vi "Main Tclk.vi"() -> ()   [LabVIEW 2018] (continued)
                    n1849 = shared-variable ".\\Zeiss Library.lvlib\\Timestamp"() -> (w7479:timestamp)  [unwired: 1 in, 1 out]
                    n1850 = Unbundle By Name(w7478) -> ("Frames"=w7475:u8, "Y tiles"=w7477:u8, "X tiles"=w7476:u8)
                    n1851 = for {
                      N: w7475 -> [_]
                      tunnel: w7479 -> [w7483]
                      tunnel: w7477 -> [w7482]
                      tunnel: w7476 -> [w7481]
                      i -> [w7480]
                      n1852 = for {
                        N: w7482 -> [_]
                        tunnel: w7481 -> [w7487]
                        tunnel: w7483 -> [w7485]
                        tunnel: w7480 -> [w7484]
                        i -> [w7486]
                        n1853 = for {
                          N: w7487 -> [_]
                          tunnel: w7486 -> [w7494]
                          tunnel: w7485 -> [w7491]
                          tunnel: w7484 -> [w7490]
                          i -> [w7493]
                          w7489 = "-" ("string")
                          w7516 = "^" ("replace string (\"\")")
                          w7496 = "_" ("string")
                          n1854 = local read "Hardware Configuration"() -> (w7526:T25)
                          n1855 = local read "File Information"() -> (w7528:T31)
                          n1856 = Format Into String(w7490) -> (resulting string=w7488:string)  [unwired: 3 in, 1 out]
                          n1857 = Format Into String(w7494) -> (resulting string=w7495:string)  [unwired: 3 in, 1 out]
                          n1858 = Format Into String(w7493) -> (resulting string=w7492:string)  [unwired: 3 in, 1 out]
                          n1859 = Unbundle By Name(w7526) -> ("Machine ID"=w7525:string)
                          n1860 = Format Date/Time String(time format string (%c)="%y-%m-%d_%H%M%S", seconds (now)=w7491) -> (date/time string=w7531:string)  [unwired: 1 out]
                          n1861 = local read "SEM Options"() -> (w7511:T27)
                          n1862 = Unbundle By Name(w7528) -> ("Sample ID"=w7513:string, "File path"=w7527:path)
                          n1863 = Format Date/Time String(time format string (%c)="Y%Y\\M%m\\D%d", seconds (now)=w7491) -> (date/time string=w7536:string)  [unwired: 1 out]
                          n1864 = xnode "Match Regular Expression"("input string"=w7525, "regular expression"="/") -> ("after match"=w7535:string)  [unwired: 4 in, 4 out]
                          n1865 = Concatenate Strings(w7535, w7496, w7531, w7496, w7488, w7489, w7495, w7489, w7492, ".dat" ("string")) -> (w7537:string)
                          n1866 = Unbundle By Name(w7511) -> ("Delete after upload"=w7510:bool)
                          n1867 = Build Path(base path=w7527, name or relative path=w7536) -> (appended path=w7533:path)
                          n1868 = Build Path(base path=w7533, name or relative path=w7537) -> (appended path=w7512:path)
                          n1869 = Path To String(path=w7512) -> (string=w7519:string)
                          n1870 = shared-variable ".\\Zeiss Library.lvlib\\Upload flags path"() -> (w7498:string)  [unwired: 1 in, 1 out]
                          n1871 = Search and Replace String(replace all?=TRUE ("replace all? (F)"), input string=w7519, search string="\\", replace string=w7516) -> (result string=w7515:string)  [unwired: 4 in, 3 out]
                          n1872 = Select(t="^delete" ("replace string (\"\")"), s=w7510, f="^keep" ("replace string (\"\")")) -> (s? t:f=w7524:string)
                          n1873 = Search and Replace String(input string=w7515, search string=":", replace string=w7516) -> (result string=w7520:string)  [unwired: 5 in, 3 out]
                          n1874 = String To Path(string=w7498) -> (path=w7497:path)
                          n1875 = Concatenate Strings(w7513, "^" ("string"), w7520, w7524) -> (w7499:string)
                          n1876 = Build Path(base path=w7497, name or relative path="Filtered") -> (appended path=w7504:path)
                          n1877 = Build Path(base path=w7497, name or relative path=w7499) -> (appended path=w7509:path)
                          n1878 = File/Directory Info(path=w7504) -> (path out=w7502:path, error out=w7503:errorcluster)  [unwired: 1 in, 5 out]
                          n1879 = File/Directory Info(path=w7509) -> (path out=w7508:path, error out=w7507:errorcluster)  [unwired: 1 in, 5 out]
                          n1880 = Unbundle By Name(w7503) -> ("status"=w7501:bool)
                          n1881 = Unbundle By Name(w7507) -> ("status"=w7506:bool)
                          n1882 = case shown="True" w7501 {
                            tunnel: w7502 -> [w7538 w7540]
                            tunnel: [w7538 w7539] -> w7500
                            frame False {
                            }
                            frame True {
                              n1883 = Create Folder(path (use dialog)=w7540) -> (created path=w7539:path)  [unwired: 2 in, 2 out]
                            }
                          }
                          n1884 = case shown="False" w7506 {
                            tunnel: w7508 -> [w7544 _]
                            tunnel: w7500 -> [w7542 _]
                            tunnel: w7499 -> [w7541 _]
                            frame False {
                              n1885 = Build Path(base path=w7542, name or relative path=w7541) -> (appended path=w7543:path)
                              n1886 = Move(source path=w7544, 10:w7543) -> ()  [unwired: 3 in, 3 out]
                            }
                            frame True {
                            }
                          }
                        }
                      }
                    }
                  }
                }
                n1887 = local write "Milling Z voltage array"(w7470) -> ()
                n1888 = Array Size(array=w7470) -> (size(s)=w7445:i32)
                n1889 = Subtract(x=w7445, y=w7444) -> (x-y=w7469:i32)
                n1890 = Max & Min(x=w7445, y=w7444) -> (min(x,y)=w7446:i32)  [unwired: 1 out]
                n1891 = Array Subset(array=w7470, index=w7469, length=w7446) -> (w7471:sgl[])
                n1892 = for {
                  N: w7446 -> [_]
                  tunnel: [w7474] -> w7447 mode=indexing
                  i -> [w7474]
                }
                n1893 = call <vilib>:"Linear Fit.vi"("Y"=w7471, "X"=w7447) -> ("slope"=w7466:dbl)  [unwired: 9 in, 4 out]
                n1894 = local read "Milling para"() -> (w7464:T35)
                n1895 = local read "FIB Scan Parameters"() -> (w7467:T32)
                n1896 = Greater Or Equal?(x=w7445, y=100.0) -> (x >= y?=w7458:bool)
                n1897 = Unbundle By Name(w7464) -> ("FIB FOV (um)"=w7463:sgl)
                n1898 = Unbundle By Name(w7467) -> ("Z size (V)"=w7465:dbl)
                n1899 = Select(t=T44."Enabled" ("Disabled"), s=w7458, f=T44."Disabled and Grayed Out" ("Disabled")) -> (s? t:f=w7457:T44)
                n1900 = Divide(x=w7466, y=w7465) -> (x/y=w7462:dbl)
                n1901 = Compound Arithmetic op=MULTIPLY(w7463, sgl -1000.0 ("value"), w7462) -> (w7452:dbl)
                "Delta Z (nm)" <- w7452
                n1902 = property on="Delta Z (nm)" class="DigNum (strict)"("DisabledEnum"=w7457) -> ()  [unwired: 2 in, 2 out]
                n1903 = local read "Delta Z array"() -> (w7454:sgl[])
                n1904 = local read "SEM Specimen I array"() -> (w7456:sgl[])
                n1905 = local read "SEM Specimen I"() -> (w7423:dbl)
                n1906 = Build Array (concatenate)(w7454, w7452) -> (w7453:dbl[])
                n1907 = local write "Delta Z array"(w7453) -> ()
                n1908 = Build Array (concatenate)(w7456, w7423) -> (w7455:dbl[])
                n1909 = local write "SEM Specimen I array"(w7455) -> ()
                n1910 = local read "3D FIB-SEM Files"() -> (w7427:path)
                n1911 = local read "SEM Scan Parameters"() -> (w7432:T26)
                n1912 = Unbundle By Name(w7432) -> ("Y tiles"=w7435:u8, "X tiles"=w7433:u8)
                n1913 = Build Array(w7435, w7433) -> (w7434:u8[])
                n1914 = Quotient & Remainder(x=w7434, y=2) -> (floor(x/y)=w7430:i32[])  [unwired: 1 out]
                n1915 = Index Array(array=w7430) -> (element #1=w7441:i32, element #2=w7442:i32)  [unwired: 2 in]
                n1916 = Format Into String(w7441) -> (resulting string=w7440:string)  [unwired: 3 in, 1 out]
                n1917 = Format Into String(w7442) -> (resulting string=w7438:string)  [unwired: 3 in, 1 out]
                n1918 = Concatenate Strings("Low res_" ("string"), w7440, "-" ("string"), w7438, ".png" ("string")) -> (w7429:string)
                n1919 = Build Path(base path=w7427, name or relative path=w7429) -> (appended path=w7426:path)
                n1920 = Build Path(base path=w7427, name or relative path="Low res.png" ("string")) -> (appended path=w7425:path)
                n1921 = Copy(9:TRUE ("overwrite (F)"), 10:w7425, 11:w7426) -> ()  [unwired: 2 in, 3 out]
              }
              frame #24 {
                n1922 = local read "SEM Scan Parameters"() -> (w7668:T26)
                n1923 = local read "Auto re-engage"() -> (w7669:bool)
                n1924 = local read "Reheat from last"() -> (w7665:bool)
                n1925 = Unbundle By Name(w7668) -> ("Pixel size (nm)"=w7667:sgl, "Y tiles"=w7661:u8, "X tiles"=w7660:u8)
                n1926 = expression code="x/1000"(w7667) -> (w7666:sgl)
                n1927 = Build Array(w7661, w7660) -> (w7663:u8[])
                n1928 = Quotient & Remainder(x=w7663, y=2) -> (floor(x/y)=w7656:i32[])  [unwired: 1 out]
                n1929 = Index Array(array=w7656) -> (element #1=w7659:i32, element #2=w7658:i32)  [unwired: 2 in]
                n1930 = local read "Low res scale tiled"() -> (w7664:dbl[][])
                n1931 = Index Array(array=w7664, index (row)=w7659, index (col)=w7658) -> (element=w7657:dbl)
                n1932 = case shown="False" w7669 {
                  tunnel: w7666 -> [_ w7714]
                  tunnel: w7657 -> [_ w7713]
                  frame False {
                    n1933 = local read "Re-engage counts"() -> (w7689:u8)
                    n1934 = local read "Last re-engage count"() -> (w7691:u8)
                    n1935 = Less?(x=w7689, y=w7691) -> (x < y?=w7690:bool)
                    n1936 = case shown="True" w7690 {
                      tunnel: w7689 -> [_ w7700]
                      tunnel: w7689 -> [_ w7701]
                      frame False {
                      }
                      frame True {
                        n1937 = local read "Delta X"() -> (w7693:sgl)
                        n1938 = local read "Re-engage X shift array"() -> (w7702:dbl[])
                        n1939 = local read "SEM Scan Parameters"() -> (w7707:T26)
                        n1940 = local read "Delta Y"() -> (w7696:sgl)
                        n1941 = local read "Re-engage Y shift array"() -> (w7703:dbl[])
                        n1942 = Decrement(x=w7701) -> (x-1=w7695:u8)
                        n1943 = Decrement(x=w7700) -> (x-1=w7698:u8)
                        n1944 = Unbundle By Name(w7707) -> ("Pixel size (nm)"=w7708:sgl)
                        n1945 = Index Array(array=w7702, index=w7695) -> (element=w7694:dbl)
                        n1946 = Index Array(array=w7703, index=w7698) -> (element=w7699:dbl)
                        n1947 = expression code="x/1000"(w7708) -> (w7705:sgl)
                        n1948 = Divide(x=w7694, y=w7705) -> (x/y=w7692:dbl)
                        n1949 = Divide(x=w7699, y=w7705) -> (x/y=w7697:dbl)
                        n1950 = Subtract(x=w7693, y=w7692) -> (x-y=w7706:dbl)
                        n1951 = Subtract(x=w7696, y=w7697) -> (x-y=w7704:dbl)
                        n1952 = local read "Re-engage Delta X array"() -> (w7712:dbl[])
                        n1953 = local read "Re-engage Delta Y array"() -> (w7709:dbl[])
                        n1954 = Build Array (concatenate)(w7712, w7706) -> (w7711:dbl[])
                        n1955 = Build Array (concatenate)(w7709, w7704) -> (w7710:dbl[])
                        n1956 = local write "Re-engage Delta X array"(w7711) -> ()
                        n1957 = local write "Re-engage Delta Y array"(w7710) -> ()
                      }
                    }
                  }
                  frame True {
                    n1958 = local read "Re-engage Files"() -> (w7715:path)
                    n1959 = stacked-sequence {
                      tunnel: w7715 -> [w7716 w7743]
                      tunnel: w7714 -> [_ w7728]
                      tunnel: w7713 -> [_ w7727]
                      frame #0 {
                        n1960 = Build Path(base path=w7716, name or relative path="post.png " ("command line")) -> (appended path=w7721:path)
                        n1961 = local read "3D FIB-SEM Files"() -> (w7719:path)
                        n1962 = Build Path(base path=w7719, name or relative path="Low res.png " ("command line")) -> (appended path=w7720:path)
                        n1963 = Copy(9:TRUE ("run minimized? (F)"), 10:w7721, 11:w7720) -> ()  [unwired: 2 in, 3 out]
                      }
                      frame #1 {
                        n1964 = local read "SEM Options"() -> (w7749:T27)
                        n1965 = Unbundle By Name(w7749) -> ("Inverse PNG"=w7748:bool)
                        n1966 = call "SIFT align.vi"("Inverse PNG"=w7748, "Affine"=TRUE, "working directory"=w7743) -> ("failed"=→"Image shift search failed":bool, "Delta Y"=w7747:dbl, "Delta X"=w7744:dbl)  [unwired: 3 in, 3 out]
                        n1967 = local read "Re-engage X shift (um)"() -> (w7742:dbl)
                        n1968 = local read "Re-engage Y shift (um)"() -> (w7745:dbl)
                        n1969 = Multiply(x=w7727, y=w7744) -> (x*y=w7739:dbl)
                        n1970 = Multiply(x=w7727, y=w7747) -> (x*y=w7729:dbl)
                        n1971 = local read "Re-engage counts"() -> (w7723:u8)
                        n1972 = Add(x=w7739, y=w7742) -> (x+y=w7740:dbl)
                        "Re-engage X shift (um)" <- w7740
                        n1973 = Add(x=w7729, y=w7745) -> (x+y=w7733:dbl)
                        "Re-engage Y shift (um)" <- w7733
                        n1974 = Greater Or Equal?(x=w7723, y=u8 2) -> (x >= y?=w7726:bool)
                        n1975 = Select(t=w7739, s=w7726, f=w7740) -> (s? t:f=w7736:dbl)
                        n1976 = Select(t=w7729, s=w7726, f=w7733) -> (s? t:f=w7734:dbl)
                        n1977 = local read "Re-engage Delta X array"() -> (w7738:dbl[])
                        n1978 = local read "Re-engage Delta Y array"() -> (w7731:dbl[])
                        n1979 = Divide(x=w7736, y=w7728) -> (x/y=w7735:dbl)
                        n1980 = Divide(x=w7734, y=w7728) -> (x/y=w7730:dbl)
                        n1981 = Greater?(x=w7723, y=u8 3) -> (0:w7724:bool)
                        n1982 = Build Array (concatenate)(w7738, w7735) -> (w7737:dbl[])
                        n1983 = Build Array (concatenate)(w7731, w7730) -> (w7732:dbl[])
                        n1984 = local write "SW error warning armed"(w7724) -> ()
                        n1985 = local write "Re-engage Delta X array"(w7737) -> ()
                        n1986 = local write "Re-engage Delta Y array"(w7732) -> ()
                      }
                    }
                  }
                }
                n1987 = case shown="True" w7665 {
                  tunnel: w7657 -> [_ w7670]
                  frame False {
                  }
                  frame True {
                    n1988 = local read "Re-engage Files"() -> (w7671:path)
                    n1989 = stacked-sequence {
                      tunnel: w7671 -> [w7678 w7685]
                      tunnel: w7670 -> [_ w7681]
                      frame #0 {
                        n1990 = Build Path(base path=w7678, name or relative path="post.png " ("command line")) -> (appended path=w7673:path)
                        n1991 = local read "3D FIB-SEM Files"() -> (w7675:path)
                        n1992 = Build Path(base path=w7675, name or relative path="Low res.png " ("command line")) -> (appended path=w7674:path)
                        n1993 = Copy(9:TRUE ("run minimized? (F)"), 10:w7673, 11:w7674) -> ()  [unwired: 2 in, 3 out]
                      }
                      frame #1 {
                        n1994 = local read "SEM Options"() -> (w7687:T27)
                        n1995 = Unbundle By Name(w7687) -> ("Inverse PNG"=w7688:bool)
                        n1996 = call "SIFT align.vi"("Inverse PNG"=w7688, "Affine"=TRUE, "working directory"=w7685) -> ("failed"=w7684:bool, "Delta Y"=w7682:dbl, "Delta X"=w7683:dbl)  [unwired: 3 in, 3 out]
                        n1997 = local write "Image shift search failed"(w7684) -> ()
                        n1998 = Multiply(x=w7681, y=w7683) -> (x*y=→"X shift from last":dbl)
                        n1999 = Multiply(x=w7681, y=w7682) -> (x*y=→"Y shift from last":dbl)
                      }
                    }
                  }
                }
              }
              frame #25 {
                w7769 = u8 2 ("y")
                n2000 = local read "Re-engage Delta X array"() -> (w7772:dbl[])
                n2001 = local read "Re-engage counts"() -> (w7770:u8)
                n2002 = local read "Re-engage Delta Y array"() -> (w7767:dbl[])
                n2003 = local read "FIB"() -> (w7776:bool)
                n2004 = local read "Delta X"() -> (w7775:sgl)
                n2005 = local read "Delta Y"() -> (w7774:sgl)
                n2006 = local read "Delta image"() -> (w7787:sgl)
                n2007 = local read "FRC resolution"() -> (w7751:sgl)
                n2008 = Subtract(x=w7770, y=w7769) -> (x-y=w7766:u8)
                n2009 = Index Array(array=w7772, index=w7766) -> (element=w7771:dbl)
                n2010 = Index Array(array=w7767, index=w7766) -> (element=w7768:dbl)
                n2011 = Greater Or Equal?(x=w7770, y=w7769) -> (x >= y?=w7773:bool)
                n2012 = Select(t=w7771, s=w7773, f=w7775) -> (s? t:f=w7757:dbl)
                n2013 = Select(t=w7768, s=w7773, f=w7774) -> (s? t:f=w7754:dbl)
                n2014 = case shown="True" w7776 {
                  tunnel: w7787 -> [_ w7858]
                  tunnel: w7757 -> [_ w7852]
                  tunnel: w7754 -> [_ w7851]
                  frame False {
                  }
                  frame True {
                    w7822 = enum16{"start", "end", "current"}."start" ("from (0:start)")
                    w7823 = enum16{"start", "end", "current"}."end" ("from (0:start)")
                    w7799 = 10000 ("count")
                    w7825 = -1 ("x")
                    w7882 = "," ("delimiter (Tab)")
                    w7880 = ".csv" ("string")
                    w7878 = T49."open" ("operation (0:open)")
                    w7879 = enum16{"start", "end", "current"}."end" ("from (0:start)")
                    n2015 = local read "File Information"() -> (w7881:T31)
                    n2016 = shared-variable ".\\Zeiss Library.lvlib\\Timestamp"() -> (w7860:timestamp)  [unwired: 1 in, 1 out]
                    n2017 = Unbundle By Name(w7881) -> ("File path"=w7861:path)
                    n2018 = Format Date/Time String(time format string (%c)="Y%Y\\%Y", seconds (now)=w7860) -> (date/time string=w7871:string)  [unwired: 1 out]
                    n2019 = Format Date/Time String(time format string (%c)="Y%Y\\M%m\\%Y-%m", seconds (now)=w7860) -> (date/time string=w7866:string)  [unwired: 1 out]
                    n2020 = Format Date/Time String(time format string (%c)="Y%Y\\M%m\\D%d\\%Y-%m-%d", seconds (now)=w7860) -> (date/time string=w7867:string)  [unwired: 1 out]
                    n2021 = Concatenate Strings(w7871, w7880) -> (w7865:string)
                    n2022 = Concatenate Strings(w7866, w7880) -> (w7864:string)
                    n2023 = Concatenate Strings(w7867, w7880) -> (w7863:string)
                    n2024 = Build Array(w7852, w7851, w7858) -> (w7884:dbl[])
                    n2025 = Build Path(base path=w7861, name or relative path=w7865) -> (appended path=w7877:path)
                    n2026 = Build Path(base path=w7861, name or relative path=w7864) -> (appended path=w7869:path)
                    n2027 = Build Path(base path=w7861, name or relative path=w7863) -> (appended path=w7862:path)
                    n2028 = Open/Create/Replace File(file path (use dialog)=w7877, operation (0:open)=w7878) -> (refnum out=w7850:refnum<file>, error out=w7849:errorcluster)  [unwired: 1 in, 4 out]
                    n2029 = Open/Create/Replace File(file path (use dialog)=w7869, operation (0:open)=w7878) -> (refnum out=w7834:refnum<file>, error out=w7833:errorcluster)  [unwired: 1 in, 4 out]
                    n2030 = local read "SEM Scan Parameters"() -> (w7797:T26)
                    n2031 = Open/Create/Replace File(file path (use dialog)=w7862, operation (0:open)=w7878) -> (refnum out=w7842:refnum<file>, error out=w7841:errorcluster)  [unwired: 1 in, 4 out]
                    n2032 = Unbundle By Name(w7797) -> ("X tiles"=w7796:u8, "Y tiles"=w7795:u8, "Frames"=w7791:u8)
                    n2033 = Compound Arithmetic op=MULTIPLY(w7796, w7795, w7791) -> (w7793:u8)
                    n2034 = expression code="2*x-1"(w7793) -> (w7794:u8)
                    n2035 = for {
                      N: 10000 -> [_]
                      tunnel: w7849 -> [w7948]
                      tunnel: w7850 -> [w7947]
                      tunnel: [w7944] -> w7848
                      tunnel: [w7943] -> w7847
                      tunnel: [w7941] -> w7845
                      tunnel: w7823 -> [w7936]
                      shift-right: [w7933] -> _
                      shift-left: u8 0 ("count") -> [w7934]
                      tunnel: w7794 -> [w7932]
                      i -> [w7939]
                      stop <- w7931 stop-if-true
                      n2036 = expression code="-x-2"(w7939) -> (w7941:i32)
                      n2037 = Set File Position(offset (in bytes) (0)=w7941, refnum=w7947, from (0:start)=w7936, error in=w7948) -> (refnum out=w7946:refnum<file>, error out=w7945:errorcluster)
                      n2038 = Read from Text File(file (use dialog)=w7946, count=w7939, error in=w7945) -> (refnum out=w7944:refnum<file>, text=w7942:string, error out=w7943:errorcluster)  [unwired: 1 in, 1 out]
                      n2039 = Match Pattern(string=w7942, regular expression="\n") -> (offset past match=w7938:i32)  [unwired: 1 in, 3 out]
                      n2040 = Equal?(x=w7938, y=1 ("x")) -> (x = y?=w7935:bool)
                      n2041 = case shown="True" w7935 {
                        tunnel: w7934 -> [w7949 w7951]
                        tunnel: [w7949 w7950] -> w7933
                        frame False {
                        }
                        frame True {
                          n2042 = Increment(x=w7951) -> (x+1=w7950:u8)
                        }
                      }
                      n2043 = Equal?(x=w7933, y=w7932) -> (x = y?=w7931:bool)
                    }
                    n2044 = expression code="x+2"(w7793) -> (w7792:u8)
                    n2045 = expression code="x-2"(w7845) -> (w7844:i32)
                    n2046 = Set File Position(offset (in bytes) (0)=w7845, refnum=w7848, from (0:start)=w7823, error in=w7847) -> (refnum out=w7856:refnum<file>, error out=w7857:errorcluster)
                    n2047 = Read from Text File(file (use dialog)=w7856, error in=w7857) -> (refnum out=w7821:refnum<file>, text=w7855:string, error out=w7820:errorcluster)  [unwired: 2 in, 1 out]
                    n2048 = Array To Spreadsheet String(delimiter (Tab)=w7882, array=w7884, 3:"%#g" ("format string")) -> (spreadsheet string=w7883:string)
                    n2049 = Set File Position(refnum=w7821, from (0:start)=w7822, error in=w7820) -> (refnum out=w7817:refnum<file>, error out=w7816:errorcluster)  [unwired: 1 in]
                    n2050 = Set File Position(refnum=w7834, from (0:start)=w7822, error in=w7833) -> (refnum out=w7807:refnum<file>, error out=w7803:errorcluster)  [unwired: 1 in]
                    n2051 = Set File Position(refnum=w7842, from (0:start)=w7822, error in=w7841) -> (refnum out=w7802:refnum<file>, error out=w7809:errorcluster)  [unwired: 1 in]
                    n2052 = Match Pattern(string=w7855, regular expression="\n") -> (after substring=w7854:string)  [unwired: 1 in, 3 out]
                    n2053 = Get File Size(file=w7817, error in=w7816) -> (refnum out=w7805:refnum<file>, size (in bytes)=w7814:i64, 0:w7815:errorcluster)
                    n2054 = Get File Size(file=w7807, error in=w7803) -> (refnum out=w7806:refnum<file>, size (in bytes)=w7812:i64, 0:w7804:errorcluster)
                    n2055 = Get File Size(file=w7802, error in=w7809) -> (refnum out=w7801:refnum<file>, size (in bytes)=w7810:i64, 0:w7800:errorcluster)
                    n2056 = Concatenate Strings(w7882, w7883, w7854) -> (w7859:string)
                    n2057 = Max & Min(x=w7799, y=w7814) -> (min(x,y)=w7813:i64)  [unwired: 1 out]
                    n2058 = Max & Min(x=w7799, y=w7812) -> (min(x,y)=w7811:i64)  [unwired: 1 out]
                    n2059 = Max & Min(x=w7799, y=w7810) -> (min(x,y)=w7808:i64)  [unwired: 1 out]
                    n2060 = Read from Text File(file (use dialog)=w7805, count=w7813, error in=w7815) -> (refnum out=w7819:refnum<file>, text=w7827:string, error out=w7818:errorcluster)  [unwired: 1 in, 1 out]
                    n2061 = Read from Text File(file (use dialog)=w7806, count=w7811, error in=w7804) -> (refnum out=w7832:refnum<file>, text=w7830:string, error out=w7831:errorcluster)  [unwired: 1 in, 1 out]
                    n2062 = Read from Text File(file (use dialog)=w7801, count=w7808, error in=w7800) -> (refnum out=w7839:refnum<file>, text=w7843:string, error out=w7838:errorcluster)  [unwired: 1 in, 1 out]
                    n2063 = for {
                      N: w7792 -> [_]
                      shift-right: [w7899] -> _
                      shift-left: w7827 -> [w7898]
                      tunnel: [w7897] -> w7826
                      n2064 = Match Pattern(string=w7898, regular expression="\n") -> (after substring=w7899:string, offset past match=w7897:i32)  [unwired: 1 in, 2 out]
                    }
                    n2065 = for {
                      N: w7792 -> [_]
                      shift-right: [w7914] -> _
                      shift-left: w7830 -> [w7913]
                      tunnel: [w7912] -> w7829
                      n2066 = Match Pattern(string=w7913, regular expression="\n") -> (after substring=w7914:string, offset past match=w7912:i32)  [unwired: 1 in, 2 out]
                    }
                    n2067 = for {
                      N: w7792 -> [_]
                      shift-right: [w7929] -> _
                      shift-left: w7843 -> [w7928]
                      tunnel: [w7927] -> w7840
                      n2068 = Match Pattern(string=w7928, regular expression="\n") -> (after substring=w7929:string, offset past match=w7927:i32)  [unwired: 1 in, 2 out]
                    }
                    n2069 = Not Equal?(x=w7825, y=w7826) -> (x != y?=w7824:bool)
                    n2070 = Not Equal?(x=w7825, y=w7829) -> (x != y?=w7828:bool)
                    n2071 = Not Equal?(x=w7825, y=w7840) -> (x != y?=w7837:bool)
                    n2072 = case shown="True" w7824 {
                      tunnel: w7879 -> [_ w7896]
                      tunnel: [w7887 w7893] -> w7876
                      tunnel: [w7886 w7892] -> w7875
                      tunnel: w7859 -> [_ w7891]
                      tunnel: w7819 -> [w7887 w7890]
                      tunnel: w7818 -> [w7886 w7889]
                      tunnel: w7844 -> [_ w7888]
                      frame False {
                      }
                      frame True {
                        n2073 = Set File Position(offset (in bytes) (0)=w7888, refnum=w7890, from (0:start)=w7896, error in=w7889) -> (refnum out=w7894:refnum<file>, error out=w7895:errorcluster)
                        n2074 = Write to Text File(file (use dialog)=w7894, text=w7891, error in=w7895) -> (refnum out=w7893:refnum<file>, error out=w7892:errorcluster)  [unwired: 2 out]
                      }
                    }
                    n2075 = case shown="False" w7828 {
                      tunnel: w7879 -> [_ w7911]
                      tunnel: [w7901 w7910] -> w7874
                      tunnel: [w7902 w7909] -> w7873
                      tunnel: w7859 -> [_ w7906]
                      tunnel: w7844 -> [_ w7905]
                      tunnel: w7832 -> [w7902 w7904]
                      tunnel: w7831 -> [w7901 w7903]
                      frame False {
                      }
                      frame True {
                        n2076 = Set File Position(offset (in bytes) (0)=w7905, refnum=w7904, from (0:start)=w7911, error in=w7903) -> (refnum out=w7908:refnum<file>, error out=w7907:errorcluster)
                        n2077 = Write to Text File(file (use dialog)=w7908, text=w7906, error in=w7907) -> (refnum out=w7909:refnum<file>, error out=w7910:errorcluster)  [unwired: 2 out]
                      }
                    }
                    n2078 = case shown="True" w7837 {
                      tunnel: w7879 -> [_ w7926]
                      tunnel: w7859 -> [_ w7924]
                      tunnel: w7844 -> [_ w7923]
                      tunnel: w7839 -> [w7917 w7921]
                      tunnel: w7838 -> [w7916 w7920]
                      tunnel: [w7917 w7919] -> w7836
                      tunnel: [w7916 w7918] -> w7835
                      frame False {
                      }
                      frame True {
                        n2079 = Set File Position(offset (in bytes) (0)=w7923, refnum=w7921, from (0:start)=w7926, error in=w7920) -> (refnum out=w7925:refnum<file>, error out=w7922:errorcluster)
                        n2080 = Write to Text File(file (use dialog)=w7925, text=w7924, error in=w7922) -> (refnum out=w7919:refnum<file>, error out=w7918:errorcluster)  [unwired: 2 out]
                      }
                    }
                    n2081 = Close File(refnum=w7876, error in=w7875) -> ()  [unwired: 2 out]
                    n2082 = Close File(refnum=w7873, error in=w7874) -> ()  [unwired: 2 out]
                    n2083 = Close File(refnum=w7836, error in=w7835) -> ()  [unwired: 2 out]
                  }
                }
                n2084 = To Single Precision Float(number=w7787) -> (single precision float=w7764:sgl)
                n2085 = local read "Delta X array"() -> (w7790:sgl[])
                n2086 = local read "Delta X sum array"() -> (w7785:sgl[])
                n2087 = local read "Delta Y array"() -> (w7788:sgl[])
                n2088 = local read "Delta Y sum array"() -> (w7778:sgl[])
                n2089 = local read "Delta image array"() -> (w7789:sgl[])
                n2090 = local read "FRC array"() -> (w7752:sgl[])
                n2091 = Build Array (concatenate)(w7790, w7757) -> (w7763:dbl[])
                n2092 = Build Array (concatenate)(w7788, w7754) -> (w7761:dbl[])
                n2093 = Array Size(array=w7785) -> (size(s)=w7786:i32)
                n2094 = Array Size(array=w7778) -> (size(s)=w7779:i32)
                n2095 = local write "Delta X array"(w7763) -> ()
                n2096 = Build Array (concatenate)(w7789, w7764) -> (w7765:sgl[])
                n2097 = Build Array (concatenate)(w7752, w7751) -> (w7753:sgl[])
                n2098 = local write "Delta Y array"(w7761) -> ()
                n2099 = Decrement(x=w7786) -> (x-1=w7784:i32)
                n2100 = Decrement(x=w7779) -> (x-1=w7780:i32)
                n2101 = local write "Delta image array"(w7765) -> ()
                n2102 = local write "FRC array"(w7753) -> ()
                n2103 = Index Array(array=w7785, index=w7784) -> (element=w7783:sgl)
                n2104 = Index Array(array=w7778, index=w7780) -> (element=w7781:sgl)
                n2105 = Add(x=w7783, y=w7757) -> (x+y=w7782:dbl)
                n2106 = Add(x=w7781, y=w7754) -> (x+y=w7777:dbl)
                n2107 = local read "Delta X array for stop limit"() -> (w7758:sgl[])
                n2108 = local read "Delta Y array for stop limit"() -> (w7755:sgl[])
                n2109 = Build Array (concatenate)(w7785, w7782) -> (w7762:dbl[])
                n2110 = Build Array (concatenate)(w7778, w7777) -> (w7760:dbl[])
                n2111 = local write "Delta X sum array"(w7762) -> ()
                n2112 = local write "Delta Y sum array"(w7760) -> ()
                n2113 = Build Array (concatenate)(w7758, w7757) -> (w7759:dbl[])
                n2114 = Build Array (concatenate)(w7755, w7754) -> (w7756:dbl[])
                n2115 = local write "Delta X array for stop limit"(w7759) -> ()
                n2116 = local write "Delta Y array for stop limit"(w7756) -> ()
              }
              frame #26 {
                n2117 = local read "Faraday Cup before mill"() -> (w7991:sgl)
                n2118 = local read "Faraday Cup array"() -> (w7988:sgl[])
                n2119 = local read "Milling para"() -> (w7986:T35)
                n2120 = local read "FIB CL control band factor"() -> (w7952:sgl)
                n2121 = Unbundle By Name(w7986) -> ("FIB PID on"=w7985:bool, "FIB PID measured"=w7984:u8, "FIB PID target"=w7956:sgl)
                n2122 = local read "FIB CL control band"() -> (w7955:sgl)
                n2123 = Array Size(array=w7988) -> (size(s)=w7990:i32)
                n2124 = Greater Or Equal?(x=w7990, y=10 ("x")) -> (x >= y?=w7987:bool)
                n2125 = Add(x=w7956, y=w7955) -> (x+y=w7954:sgl)
                n2126 = Subtract(x=w7956, y=w7955) -> (x-y=w7953:sgl)
                n2127 = case shown="True" w7987 {
                  tunnel: w7991 -> [w8324 w8328]
                  tunnel: w7988 -> [_ w8339]
                  tunnel: [w8317 w8337] -> _
                  tunnel: [w8317 w8326] -> w7983
                  frame False {
                    w8325 = sgl 0.5 ("y")
                    w8317 = FALSE
                    n2128 = local read "Faraday Cup low limit array"() -> (w8322:sgl[])
                    n2129 = local read "Faraday Cup high limit array"() -> (w8320:sgl[])
                    n2130 = Subtract(x=w8324, y=w8325) -> (x-y=w8321:sgl)
                    n2131 = Add(x=w8325, y=w8324) -> (x+y=w8318:sgl)
                    n2132 = Build Array (concatenate)(w8322, w8321) -> (w8323:sgl[])
                    n2133 = Build Array (concatenate)(w8320, w8318) -> (w8319:sgl[])
                    n2134 = local write "Faraday Cup low limit array"(w8323) -> ()
                    n2135 = local write "Faraday Cup high limit array"(w8319) -> ()
                  }
                  frame True {
                    n2136 = call "Auto limits.vi"("Minimum half range"=0.5, "# of interquartile range or stdev"=6.0 ("# of sigma"), "Length"=1000, "Input array"=w8339) -> ("Low limit"=w8327:dbl, "High limit"=w8334:dbl)  [unwired: 5 in, 1 out]
                    n2137 = Less Or Equal?(x=w8328, y=w8327) -> (x <= y?=w8326:bool)
                    n2138 = local read "Faraday Cup high limit array"() -> (w8335:sgl[])
                    n2139 = local read "Faraday Cup low limit array"() -> (w8331:sgl[])
                    n2140 = To Single Precision Float(number=w8334) -> (single precision float=w8329:sgl)
                    n2141 = To Single Precision Float(number=w8327) -> (single precision float=w8330:sgl)
                    n2142 = In Range and Coerce(upper limit=w8329, x=w8328, lower limit=w8330) -> (In Range?=w8338:bool)  [unwired: 1 out]
                    n2143 = Build Array (concatenate)(w8335, w8329) -> (w8333:sgl[])
                    n2144 = Build Array (concatenate)(w8331, w8330) -> (w8332:sgl[])
                    n2145 = Not(x=w8338) -> (.not. x?=w8337:bool)
                    n2146 = local write "Faraday Cup high limit array"(w8333) -> ()
                    n2147 = local write "Faraday Cup low limit array"(w8332) -> ()
                  }
                }
                "Faraday cup I low" <- w7983
                n2148 = case shown="True" w7985 {
                  tunnel: w7984 -> [_ w8043]
                  tunnel: w7954 -> [_ w8042]
                  tunnel: w7953 -> [_ w8041]
                  tunnel: w7952 -> [_ w8040]
                  frame False {
                    n2149 = local read "Specimen I array"() -> (w8036:sgl[])
                    n2150 = local read "Beam Dump 1 array"() -> (w8019:sgl[])
                    n2151 = local read "Beam Dump 2 array"() -> (w8012:sgl[])
                    n2152 = local read "Milling I array"() -> (w7995:sgl[])
                    n2153 = call "Auto limits.vi"("Minimum half range"=0.5, "# of interquartile range or stdev"=6.0 ("# of sigma"), "Length"=100, "Input array"=w8036) -> ("Low limit"=w8034:dbl, "High limit"=w8035:dbl)  [unwired: 5 in, 1 out]
                    n2154 = call "Auto limits.vi"("Minimum half range"=0.5, "# of interquartile range or stdev"=6.0 ("# of sigma"), "Length"=100, "Input array"=w8019) -> ("Low limit"=w8021:dbl, "High limit"=w8020:dbl)  [unwired: 5 in, 1 out]
                    n2155 = call "Auto limits.vi"("Minimum half range"=0.5, "# of interquartile range or stdev"=6.0 ("# of sigma"), "Length"=100, "Input array"=w8012) -> ("Low limit"=w8010:dbl, "High limit"=w8011:dbl)  [unwired: 5 in, 1 out]
                    n2156 = call "Auto limits.vi"("Minimum half range"=0.5, "# of interquartile range or stdev"=6.0 ("# of sigma"), "Length"=100, "Input array"=w7995) -> ("Low limit"=w7997:dbl, "High limit"=w7996:dbl)  [unwired: 5 in, 1 out]
                    n2157 = To Single Precision Float(number=w8035) -> (single precision float=w8029:sgl)
                    n2158 = To Single Precision Float(number=w8034) -> (single precision float=w8028:sgl)
                    n2159 = To Single Precision Float(number=w8020) -> (single precision float=w8026:sgl)
                    n2160 = To Single Precision Float(number=w8021) -> (single precision float=w8027:sgl)
                    n2161 = To Single Precision Float(number=w8011) -> (single precision float=w8005:sgl)
                    n2162 = To Single Precision Float(number=w8010) -> (single precision float=w8004:sgl)
                    n2163 = To Single Precision Float(number=w7996) -> (single precision float=w8002:sgl)
                    n2164 = To Single Precision Float(number=w7997) -> (single precision float=w8003:sgl)
                    n2165 = local read "Specimen I high limit array"() -> (w8031:sgl[])
                    n2166 = local read "Specimen I low limit array"() -> (w8032:sgl[])
                    n2167 = local read "BD1 high limit array"() -> (w8024:sgl[])
                    n2168 = local read "BD2 high limit array"() -> (w8007:sgl[])
                    n2169 = local read "Milling I high limit array"() -> (w8000:sgl[])
                    n2170 = local read "BD1 low limit array"() -> (w8023:sgl[])
                    n2171 = local read "BD2 low limit array"() -> (w8008:sgl[])
                    n2172 = local read "Milling I low limit array"() -> (w7999:sgl[])
                    n2173 = Build Array (concatenate)(w8031, w8029) -> (w8030:sgl[])
                    n2174 = Build Array (concatenate)(w8032, w8028) -> (w8033:sgl[])
                    n2175 = Build Array (concatenate)(w8024, w8026) -> (w8025:sgl[])
                    n2176 = Build Array (concatenate)(w8023, w8027) -> (w8022:sgl[])
                    n2177 = Build Array (concatenate)(w8007, w8005) -> (w8006:sgl[])
                    n2178 = Build Array (concatenate)(w8008, w8004) -> (w8009:sgl[])
                    n2179 = Build Array (concatenate)(w8000, w8002) -> (w8001:sgl[])
                    n2180 = Build Array (concatenate)(w7999, w8003) -> (w7998:sgl[])
                    n2181 = local write "Specimen I high limit array"(w8030) -> ()
                    n2182 = local write "Specimen I low limit array"(w8033) -> ()
                    n2183 = local write "BD1 high limit array"(w8025) -> ()
                    n2184 = local write "BD2 high limit array"(w8006) -> ()
                    n2185 = local write "Milling I high limit array"(w8001) -> ()
                    n2186 = local write "BD1 low limit array"(w8022) -> ()
                    n2187 = local write "BD2 low limit array"(w8009) -> ()
                    n2188 = local write "Milling I low limit array"(w7998) -> ()
                  }
                  frame True {
                    n2189 = case shown="3" w8043 {
                      tunnel: w8042 -> [w8065 w8108 w8167 w8231 _]
                      tunnel: w8041 -> [w8064 w8107 w8166 w8230 _]
                      tunnel: w8040 -> [_ _ _ w8212 _]
                      frame 0 {
                        n2190 = local read "Specimen I (nA)"() -> (w8061:sgl)
                        n2191 = local read "Beam Dump 1 array"() -> (w8093:sgl[])
                        n2192 = local read "Beam Dump 1 (nA)"() -> (w8056:sgl)
                        n2193 = local read "Beam Dump 2 array"() -> (w8086:sgl[])
                        n2194 = local read "Beam Dump 2 (nA)"() -> (w8053:sgl)
                        n2195 = local read "Milling I array"() -> (w8073:sgl[])
                        n2196 = local read "Milling I (nA)"() -> (w8044:sgl)
                        n2197 = call "Auto limits.vi"("Minimum half range"=0.5, "# of interquartile range or stdev"=6.0 ("# of sigma"), "Length"=100, "Input array"=w8093) -> ("Low limit"=w8095:dbl, "High limit"=w8094:dbl)  [unwired: 5 in, 1 out]
                        n2198 = call "Auto limits.vi"("Minimum half range"=0.5, "# of interquartile range or stdev"=6.0 ("# of sigma"), "Length"=100, "Input array"=w8086) -> ("Low limit"=w8084:dbl, "High limit"=w8085:dbl)  [unwired: 5 in, 1 out]
                        n2199 = call "Auto limits.vi"("Minimum half range"=0.5, "# of interquartile range or stdev"=6.0 ("# of sigma"), "Length"=100, "Input array"=w8073) -> ("Low limit"=w8075:dbl, "High limit"=w8074:dbl)  [unwired: 5 in, 1 out]
                        n2200 = To Single Precision Float(number=w8065) -> (single precision float=w8060:sgl)
                        n2201 = To Single Precision Float(number=w8064) -> (single precision float=w8059:sgl)
                        n2202 = To Single Precision Float(number=w8094) -> (single precision float=w8050:sgl)
                        n2203 = To Single Precision Float(number=w8095) -> (single precision float=w8049:sgl)
                        n2204 = To Single Precision Float(number=w8085) -> (single precision float=w8052:sgl)
                        n2205 = To Single Precision Float(number=w8084) -> (single precision float=w8051:sgl)
                        n2206 = To Single Precision Float(number=w8074) -> (single precision float=w8045:sgl)
                        n2207 = To Single Precision Float(number=w8075) -> (single precision float=w8046:sgl)
                        n2208 = local read "Specimen I high limit array"() -> (w8067:sgl[])
                        n2209 = local read "Specimen I low limit array"() -> (w8068:sgl[])
                        n2210 = local read "BD1 high limit array"() -> (w8098:sgl[])
                        n2211 = local read "BD2 high limit array"() -> (w8081:sgl[])
                        n2212 = local read "Milling I high limit array"() -> (w8078:sgl[])
                        n2213 = local read "BD1 low limit array"() -> (w8097:sgl[])
                        n2214 = local read "BD2 low limit array"() -> (w8082:sgl[])
                        n2215 = local read "Milling I low limit array"() -> (w8077:sgl[])
                        n2216 = Build Array (concatenate)(w8067, w8060) -> (w8066:sgl[])
                        n2217 = In Range and Coerce(upper limit=w8060, x=w8061, lower limit=w8059) -> (In Range?=w8063:bool)  [unwired: 1 out]
                        n2218 = Build Array (concatenate)(w8068, w8059) -> (w8069:sgl[])
                        n2219 = Build Array (concatenate)(w8098, w8050) -> (w8099:sgl[])
                        n2220 = In Range and Coerce(upper limit=w8050, x=w8056, lower limit=w8049) -> (In Range?=w8057:bool)  [unwired: 1 out]
                        n2221 = Build Array (concatenate)(w8097, w8049) -> (w8096:sgl[])
                        n2222 = Build Array (concatenate)(w8081, w8052) -> (w8080:sgl[])
                        n2223 = In Range and Coerce(upper limit=w8052, x=w8053, lower limit=w8051) -> (In Range?=w8055:bool)  [unwired: 1 out]
                        n2224 = Build Array (concatenate)(w8082, w8051) -> (w8083:sgl[])
                        n2225 = Build Array (concatenate)(w8078, w8045) -> (w8079:sgl[])
                        n2226 = In Range and Coerce(upper limit=w8045, x=w8044, lower limit=w8046) -> (In Range?=w8048:bool)  [unwired: 1 out]
                        n2227 = Build Array (concatenate)(w8077, w8046) -> (w8076:sgl[])
                        n2228 = Not(x=w8063) -> (.not. x?=w8062:bool)
                        n2229 = Not(x=w8057) -> (.not. x?=w8058:bool)
                        n2230 = Not(x=w8055) -> (.not. x?=w8054:bool)
                        n2231 = Not(x=w8048) -> (.not. x?=w8047:bool)
                        n2232 = local write "Specimen I high limit array"(w8066) -> ()
                        n2233 = local write "Specimen I low limit array"(w8069) -> ()
                        n2234 = local write "BD1 high limit array"(w8099) -> ()
                        n2235 = local write "BD2 high limit array"(w8080) -> ()
                        n2236 = local write "Milling I high limit array"(w8079) -> ()
                        n2237 = local write "BD1 low limit array"(w8096) -> ()
                        n2238 = local write "BD2 low limit array"(w8083) -> ()
                        n2239 = local write "Milling I low limit array"(w8076) -> ()
                        n2240 = local write "Specimen I out of bound"(w8062) -> ()
                        n2241 = local write "BD1 out of bound"(w8058) -> ()
                        n2242 = local write "BD2 out of bound"(w8054) -> ()
                        n2243 = local write "Milling I out of bound"(w8047) -> ()
                      }
                      frame 1 {
                        n2244 = local read "Specimen I array"() -> (w8152:sgl[])
                        n2245 = local read "Specimen I (nA)"() -> (w8100:sgl)
                        n2246 = local read "Beam Dump 1 (nA)"() -> (w8103:sgl)
                        n2247 = local read "Beam Dump 2 array"() -> (w8142:sgl[])
                        n2248 = local read "Beam Dump 2 (nA)"() -> (w8102:sgl)
                        n2249 = local read "Milling I array"() -> (w8129:sgl[])
                        n2250 = local read "Milling I (nA)"() -> (w8101:sgl)
                        n2251 = call "Auto limits.vi"("Minimum half range"=0.5, "# of interquartile range or stdev"=6.0 ("# of sigma"), "Length"=100, "Input array"=w8152) -> ("Low limit"=w8150:dbl, "High limit"=w8151:dbl)  [unwired: 5 in, 1 out]
                        n2252 = call "Auto limits.vi"("Minimum half range"=0.5, "# of interquartile range or stdev"=6.0 ("# of sigma"), "Length"=100, "Input array"=w8142) -> ("Low limit"=w8140:dbl, "High limit"=w8141:dbl)  [unwired: 5 in, 1 out]
                        n2253 = call "Auto limits.vi"("Minimum half range"=0.5, "# of interquartile range or stdev"=6.0 ("# of sigma"), "Length"=100, "Input array"=w8129) -> ("Low limit"=w8131:dbl, "High limit"=w8130:dbl)  [unwired: 5 in, 1 out]
                        n2254 = To Single Precision Float(number=w8151) -> (single precision float=w8123:sgl)
                        n2255 = To Single Precision Float(number=w8150) -> (single precision float=w8122:sgl)
                        n2256 = To Single Precision Float(number=w8108) -> (single precision float=w8105:sgl)
                        n2257 = To Single Precision Float(number=w8107) -> (single precision float=w8104:sgl)
                        n2258 = To Single Precision Float(number=w8141) -> (single precision float=w8119:sgl)
                        n2259 = To Single Precision Float(number=w8140) -> (single precision float=w8118:sgl)
                        n2260 = To Single Precision Float(number=w8130) -> (single precision float=w8115:sgl)
                        n2261 = To Single Precision Float(number=w8131) -> (single precision float=w8114:sgl)
                        n2262 = local read "Specimen I high limit array"() -> (w8147:sgl[])
                        n2263 = local read "Specimen I low limit array"() -> (w8148:sgl[])
                        n2264 = local read "BD1 high limit array"() -> (w8106:sgl[])
